vi "RxTx.vi"(0 "State-machine Local Variables":T1={"Message"="", "Homed?"=FALSE, "NextState"=enum."Timeout", "G.Load"=0.0, "G.Position"=0.0, "Load#"=0, "[G.Loads]"=[], "[TotalLoads]"=[], "[Errors]"=[], "ZeroWait"=0, "Results"=[], "DwellWait"=FALSE, "Test Result"=FALSE, "[CondyleLoads]"=[], "[Max]"=[], "[Min]"=[], "Valid String?"=FALSE, "ScanTime"=timestamp(0 s since 1904-01-01), "ScannedString"="", "LabelDevID"=0, "MfgDate"=timestamp(0 s since 1904-01-01), "[EEPROM Cmds]"=[], "[CalData]"=[], "[A/Ds]"=[], "[A/Dmax]"=[], "[A/Dmin]"=[], "BattMax"=0.0, "BattMin"=0.0, "DwellTime"=2000, "PendingDeviceType"="", "Zero G.load"=0.0, "GAINC Value"="", "Programming Step"=enum."Load EEPROM", "Front Panel Program?"=FALSE, "Final Program?"=FALSE, "PCB Score"=100, "AssyScore"=100, "Pass/Fail #"="", "Result String"="", "Programming Mode"=enum."Initial Program", "Angle Test Step"=enum."Initialize", "Accel Values"=[], "Shutdown Counter"=0, "V1"=0, "V2"=0, "V3"=0, "V4"=0, "EEPROM Data"=[], "Counter"=0, "Page#"=0, "Timer"=timestamp(0 s since 1904-01-01), "Use Mark10?"=FALSE, "Eng-Result#"=0, "DUT Serial #"=0, "Scroll Message?"=FALSE, "Clear Message"=FALSE, "Batt Test Step "=enum."Initialize", "RXTX Window Found?"=FALSE, "Shutdown First Call?"=FALSE, "A2 Delay (msec)"=500, "Support Script"={"Script #"="", "Script Revision"="", "[OEMs]"=[], "[[DeviceTypes]]"=[], "[[DeviceTypesVals]]"=[], "[[List of Errors]]"=[], "Default GAINC"="", "[[ASICtrims]]"=[], "ID For Echo"="", "Condyle A CalFactor"=100, "Condyle B CalFactor"=100, "[OEMs Prefix]"=[], "Packet ID 18"="", "[[Force Table Load Test]]"=[], "[[Force Table AccurTest]]"=[]}, "Serial Table"={"Serial File Path"=path "", "[[Serial Lookup Table]]"=[], "Serial Device Info"=[], "Valid Serial?"=FALSE}, "Target Information"={"Target Brand"="", "Target DeviceType"="", "Target Serial#"=100, "Target Lot#"=0, "Target DevID"=0, "Target Channel"=5}, "Operator"="", "COM Port"="", "Config Path"=path "", "Tx Array"=[], "DUT Parameters"={"Channel"=0, "DeviceID"=0, "Script Rev"=0, "Month"=0, "Day"=0, "Year"=0, "Lot#"=0, "V1"=0, "V2"=0, "V3"=0, "V4"=0, "MFG"=0, "Cal FactorA 10"=0, "Cal FactorB 10  "=0, "Cal FactorA 16"=0, "Cal FactorB 16"=0, "ASICtrim"=[], "TmpChan"=0, "GAINC"="", "Brand"="", "Device"="", "Serial #"=0, "Batt310"=0, "Batt 280"=0}, "FTS Main?"=FALSE, "Loading"={"[Forces]"=[], "[Dwell]"=[], "Loading Step"=enum."Initialize Test"}, "Software Version"="", "Correction Factor"="", "Second Load Test"=FALSE, "Acc Loads"=[], "Mark10 Config"={"H2S%"=[80.0, 85.0, 90.0, 95.0, 100.0], "H2S Speed"=[12.0, 8.0, 6.0, 4.0, 2.0], "H to S"=2.0, "Home Speed"=1.0, "LoadWin"=0.0, "Load Speed"=0.0, "PID"={"Kp"=0.04, "Kd"=0.005001, "Ki"=2.9999999999999923e-05}}, "Channels"={"Transceiver Ch"=5, "Operating Ch"=5, "Start Ch"=0}, "Channel EEPROM"=[], "Load Notes"=[], "Engr Log?"=FALSE, "Time"=[], "Program Retry"=FALSE, "Operator Channel"="", "Target Channel "="", "New Data Program"=FALSE, "NFHU Pass?"=FALSE, "Cycle Number"=0, "Cal Cycle#"=0, "[Avg G.Loads] "=[], "[Avg A/Ds] "=[], "Cal Retry?"=FALSE, "[Total A/Ds]  "=[], "Cycle Num LA"=0, "LA Cycle# "=0, "Shim Num"=0, "Shim#  "=0, "Angle Test?"=FALSE} {"Mark10 Config"."PID"."Ki" min=0.0 max=200.0 format="%.6f"; "Mark10 Config"."PID"."Kd" min=0.0 max=200.0 format="%.6f"; "Mark10 Config"."PID"."Kp" min=0.0 max=200.0 format="%.6f"; "DUT Parameters"."ASICtrim" format="%02x"}, 2 "[TxData]":u8[](array[numeric]), 5 "error in (no error)":errorcluster, 9 "Action":T15) -> (8 "NoData?":bool, 10 "Blank?":bool, 11 "return type":i32, 14 "[Raw RxData]":u8[](array[numeric]), 15 "Alive?":bool, 16 "Stop?":bool, 17 "NewData?":bool, 18 "DUT Serial Number":u32, 19 "error out":errorcluster)   [LabVIEW 2015]
uses:
  XceiverStates.ctl
  Controls/LocalVars.ctl
  Controls/Gen2 FT states.ctl
  Controls/Iniial Device Programming.ctl
  SubVI/ProgramStageControl.ctl
  Controls/Batt Cap Steps.ctl
  Controls/Support Script.ctl
  Controls/Serial Table.ctl
  Controls/Device Information.ctl
  Controls/InfoPacket.ctl
  Controls/Loading.ctl
  Controls/Load Step.ctl
  Controls/Mark10 Config.ctl
  Controls/PID parameters.ctl
  Controls/Channels.ctl
  Controls/Gen2 FT Globals.vi
  data/SiUSBXp.dll
panel:
  out "Handle":u32
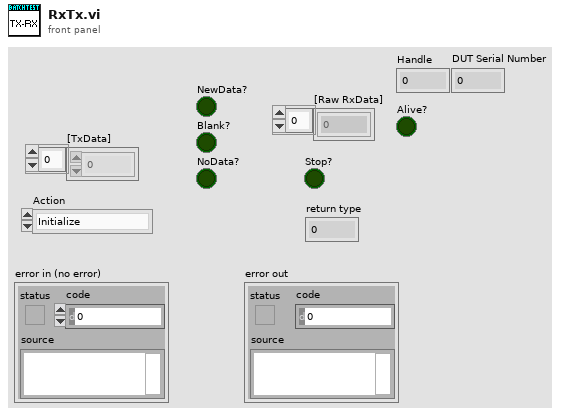
[diagram p1: front panel]
types:
  T1 = typedef "LocalVars.ctl" = cluster{"Message":string, "Homed?":bool, "NextState":T2, "G.Load":dbl, "G.Position":dbl, "Load#":i32, "[G.Loads]":dbl[], "[TotalLoads]":dbl[], "[Errors]":dbl[][], "ZeroWait":u32, "Results":dbl[], "DwellWait":bool, "Test Result":bool, "[CondyleLoads]":dbl[][], "[Max]":dbl[], "[Min]":dbl[], "Valid String?":bool, "ScanTime":timestamp, "ScannedString":string, "LabelDevID":u32, "MfgDate":timestamp, "[EEPROM Cmds]":u8[][], "[CalData]":u8[][], "[A/Ds]":dbl[][], "[A/Dmax]":dbl[], "[A/Dmin]":dbl[], "BattMax":dbl, "BattMin":dbl, "DwellTime":i32, "PendingDeviceType":string, "Zero G.load":dbl, "GAINC Value":string, "Programming Step":T3, "Front Panel Program?":bool, "Final Program?":bool, "PCB Score":i32, "AssyScore":i32, "Pass/Fail #":string, "Result String":string, "Programming Mode":T4, "Angle Test Step":enum16{"Initialize", "Get X", "Get Y", "Get Z", "Next Test"}, "Accel Values":dbl[][], "Shutdown Counter":u32, "V1":i32, "V2":i32, "V3":i32, "V4":i32, "EEPROM Data":i32[][], "Counter":i32, "Page#":i32, "Timer":timestamp, "Use Mark10?":bool, "Eng-Result#":u32, "DUT Serial #":i32, "Scroll Message?":bool, "Clear Message":bool, "Batt Test Step ":T5, "RXTX Window Found?":bool, "Shutdown First Call?":bool, "A2 Delay (msec)":i16, "Support Script":T6, "Serial Table":T7, "Target Information":T8, "Operator":string, "COM Port":string, "Config Path":path, "Tx Array":u8[], "DUT Parameters":T9, "FTS Main?":bool, "Loading":T10, "Software Version":string, "Correction Factor":string, "Second Load Test":bool, "Acc Loads":dbl[][], "Mark10 Config":T12, "Channels":T14, "Channel EEPROM":i32[][], "Load Notes":string[], "Engr Log?":bool, "Time":timestamp[], "Program Retry":bool, "Operator Channel":string, "Target Channel ":string, "New Data Program":bool, "NFHU Pass?":bool, "Cycle Number":i32, "Cal Cycle#":i32, "[Avg G.Loads] ":dbl[], "[Avg A/Ds] ":dbl[][], "Cal Retry?":bool, "[Total A/Ds]  ":dbl[][], "Cycle Num LA":i32, "LA Cycle# ":i32, "Shim Num":i32, "Shim#  ":i32, "Angle Test?":bool}
  T2 = typedef "Gen2 FT states.ctl" = enum16{"---------SETUP-------", "Initialization", "Read Support Data", "Initialize Mark-10", "Initialize Transceiver", "------UTILITIES------", "Change DUT Channel", "Find RxTx Window", "Reset Device", "Scan Channels", "Read Serial Lookup", "Shutdown Device", "ESTOP", "--------USER---------", "Timeout", "-----PROGRAM-----", "Program Device", "------MARK10--------", "Go Home", "MoveUp", "MoveDown", "Goto Load", "Goto Position", "Stop Motor", "---------TESTS--------", "Start Test", "Angle Test", "Load Test", "Load Accuracy Test", "Battery Test", "------RESULTS-------", "End Test", "Display Result", "--------EXIT--------", "Exit"}
  T3 = typedef "Iniial Device Programming.ctl" = enum16{"Load EEPROM", "Send First A1", "Send EEPROM", "Send A1", "Check EEPROM Echo", "Verify transmission", "Programming Successful", "Programming Failed"}
  T4 = typedef "ProgramStageControl.ctl" = enum16{"Initial Program", "GainC", "Scales"}
  T5 = typedef "Batt Cap Steps.ctl" = enum16{"Initialize", "Collect 2.8 Volts", "Collect 3.1 Volts", "Check Results"}
  T6 = typedef "Support Script.ctl" = cluster{"Script #":string, "Script Revision":string, "[OEMs]":string[], "[[DeviceTypes]]":string[][], "[[DeviceTypesVals]]":u16[][], "[[List of Errors]]":string[][], "Default GAINC":string, "[[ASICtrims]]":u8[][], "ID For Echo":string, "Condyle A CalFactor":i32, "Condyle B CalFactor":i32, "[OEMs Prefix]":string[], "Packet ID 18":string, "[[Force Table Load Test]]":dbl[][], "[[Force Table AccurTest]]":dbl[][]}
  T7 = typedef "Serial Table.ctl" = cluster{"Serial File Path":path, "[[Serial Lookup Table]]":string[][], "Serial Device Info":string[], "Valid Serial?":bool}
  T8 = typedef "Device Information.ctl" = cluster{"Target Brand":string, "Target DeviceType":string, "Target Serial#":i32, "Target Lot#":u32, "Target DevID":u32, "Target Channel":u8}
  T9 = typedef "InfoPacket.ctl" = cluster{"Channel":u8, "DeviceID":u32, "Script Rev":u8, "Month":u8, "Day":u8, "Year":u8, "Lot#":u32, "V1":u16, "V2":u16, "V3":u16, "V4":u16, "MFG":u8, "Cal FactorA 10":u8, "Cal FactorB 10  ":u8, "Cal FactorA 16":u8, "Cal FactorB 16":u8, "ASICtrim":u8[], "TmpChan":u8, "GAINC":string, "Brand":string, "Device":string, "Serial #":u64, "Batt310":u16, "Batt 280":u16}
  T10 = typedef "Loading.ctl" = cluster{"[Forces]":dbl[], "[Dwell]":dbl[], "Loading Step":T11}
  T11 = typedef "Load Step.ctl" = enum16{"Initialize Test", "Go Home", "Detect Dev Surface", "Wait to zero Device", "Zero Device", "Do Test", "Test Result"}
  T12 = typedef "Mark10 Config.ctl" = cluster{"H2S%":dbl[], "H2S Speed":dbl[], "H to S":dbl, "Home Speed":dbl, "LoadWin":dbl, "Load Speed":dbl, "PID":T13}
  T13 = typedef "PID parameters.ctl" = cluster{"Kp":dbl, "Kd":dbl, "Ki":dbl}
  T14 = typedef "Channels.ctl" = cluster{"Transceiver Ch":u8, "Operating Ch":u8, "Start Ch":u8}
  T15 = typedef "XceiverStates.ctl" = enum16{"Initialize", "Rx", "Tx", "Raw Mode", "Clear Buffer", "ClearEcho", "Read Buffer", "Close"}
  T16 = cluster{"Handle":u32, "TempRxData":u8[], "OffTimer":u32, "Echo?":bool, "NoData?":bool, "Alive?":bool, "Counter":u32}
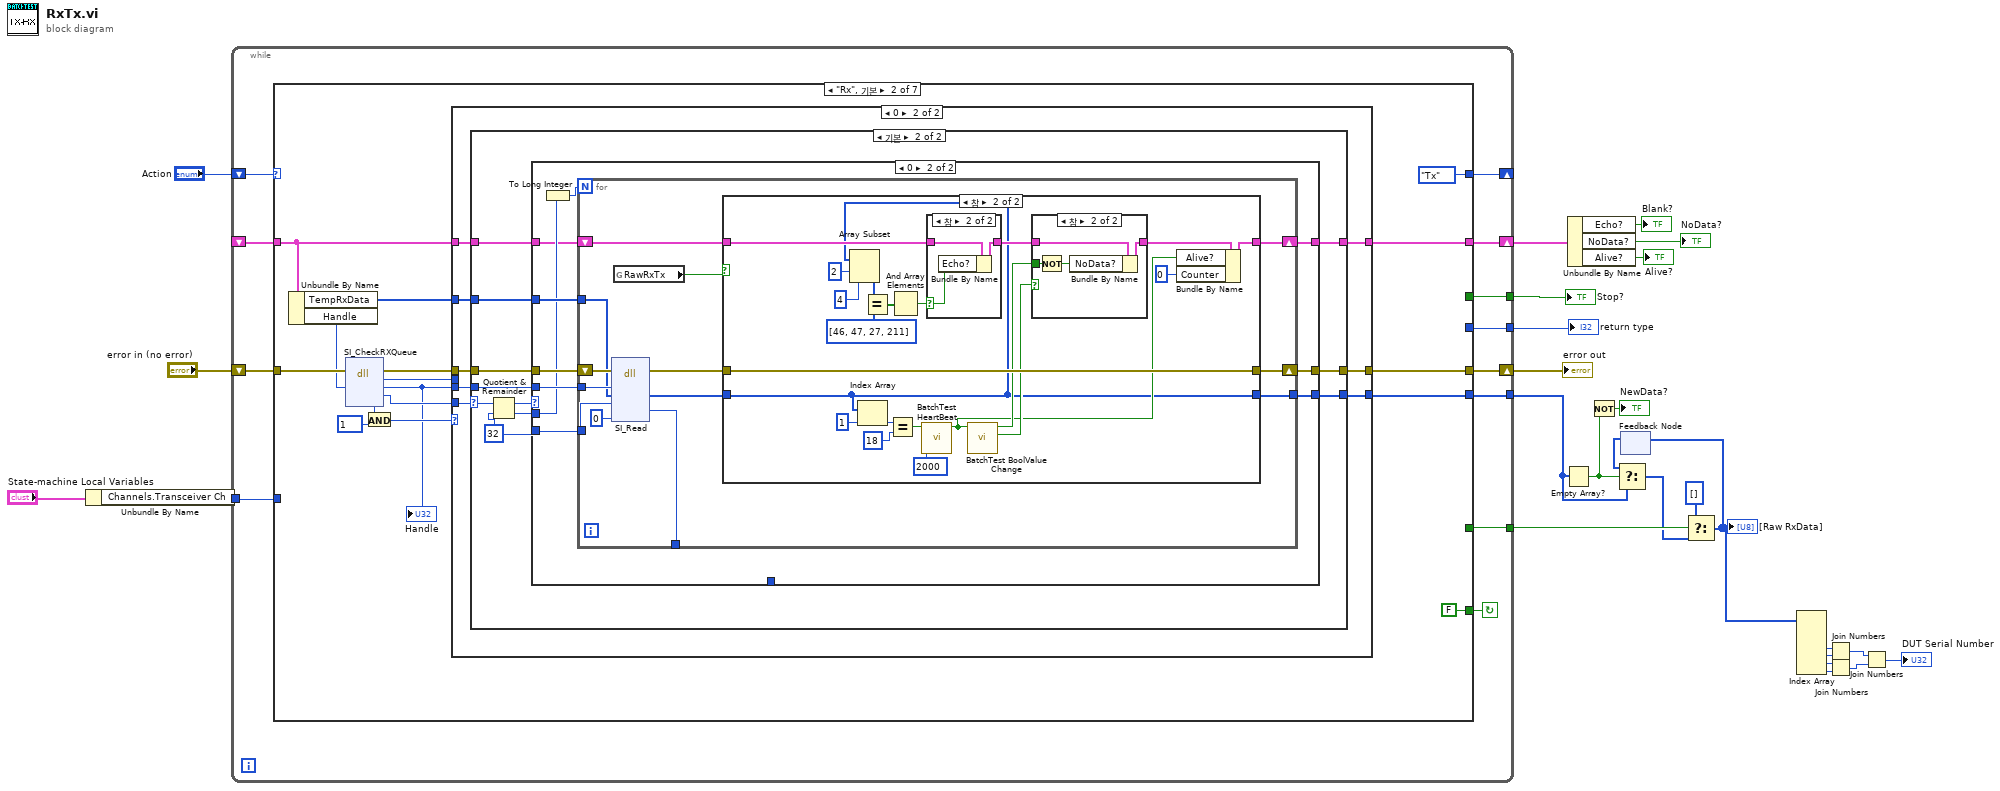
[diagram p0: block diagram]
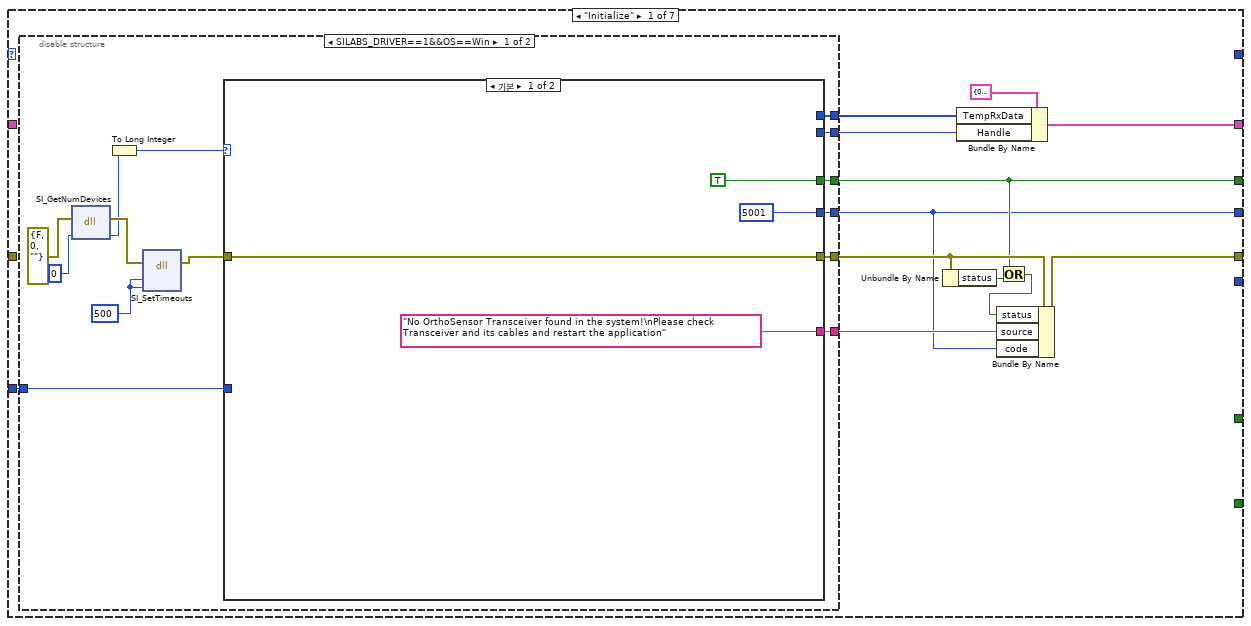
[diagram p2: hidden frame]
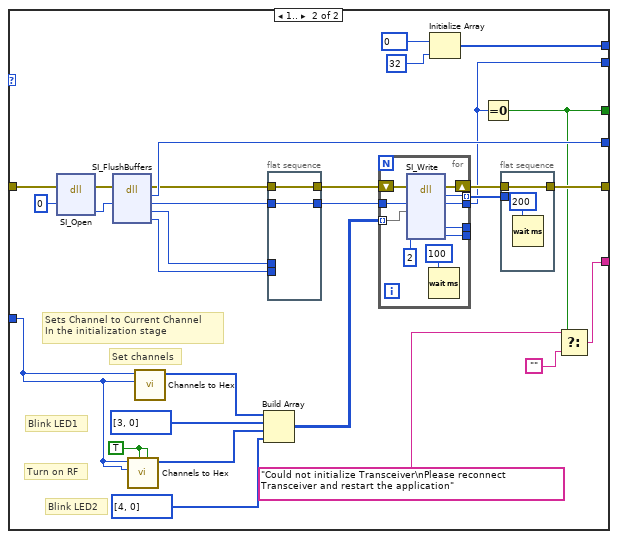
[diagram p3: hidden frame]
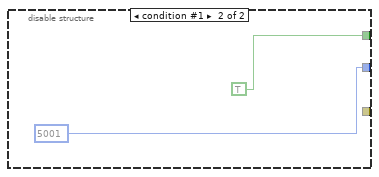
[diagram p4: hidden frame]
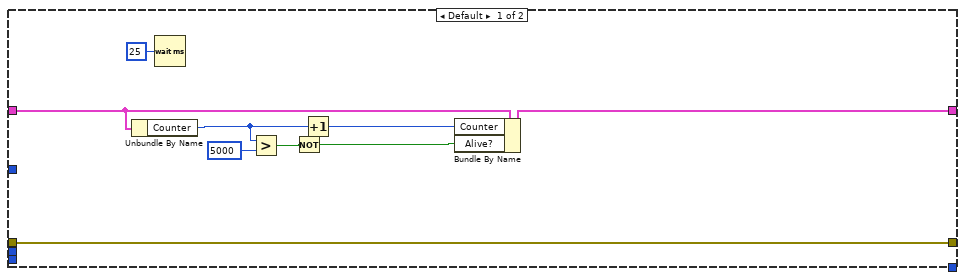
[diagram p5: hidden frame]
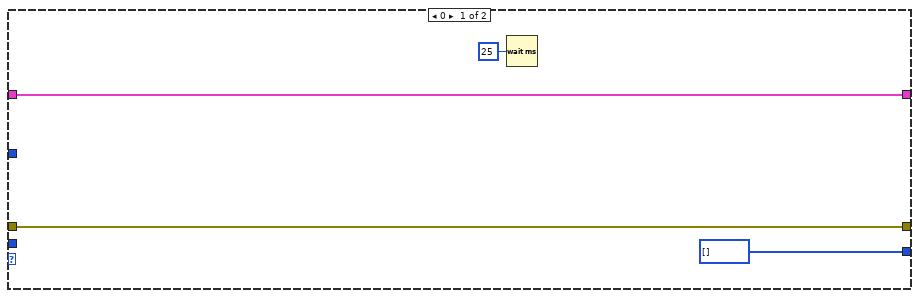
[diagram p6: hidden frame]
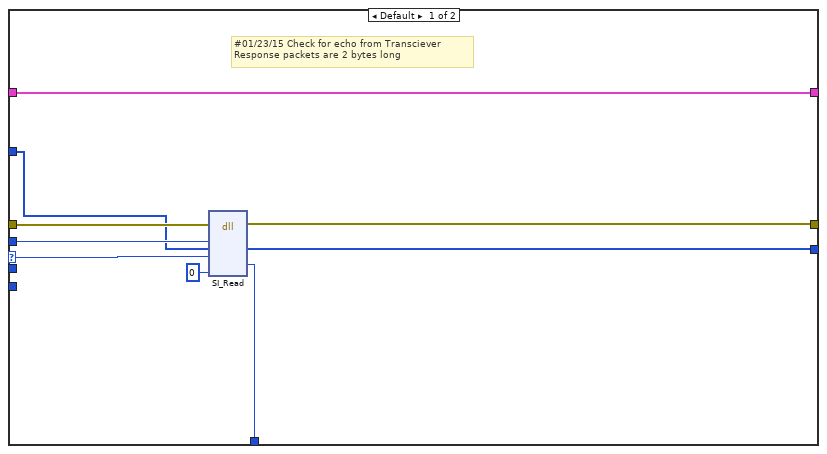
[diagram p7: hidden frame]
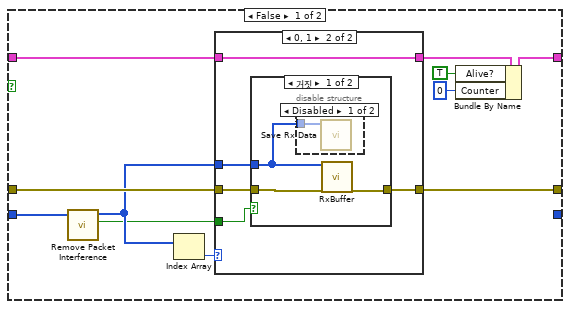
[diagram p8: hidden frame]
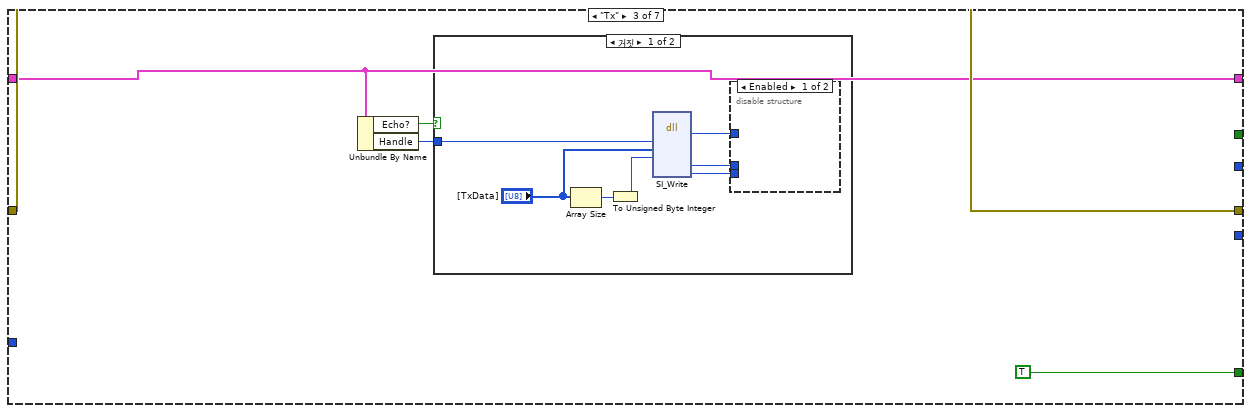
[diagram p14: hidden frame]
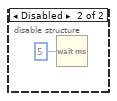
[diagram p15: hidden frame]
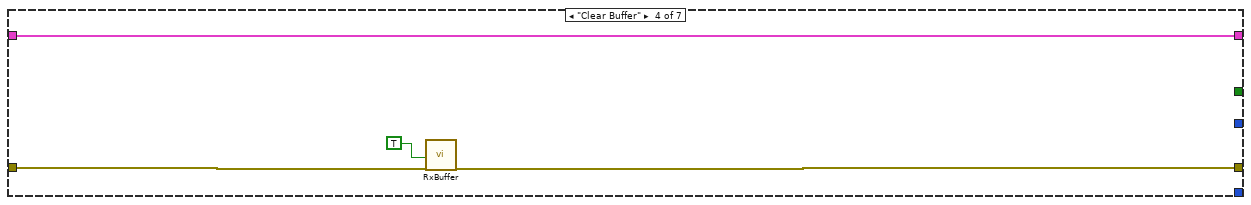
[diagram p17: hidden frame]
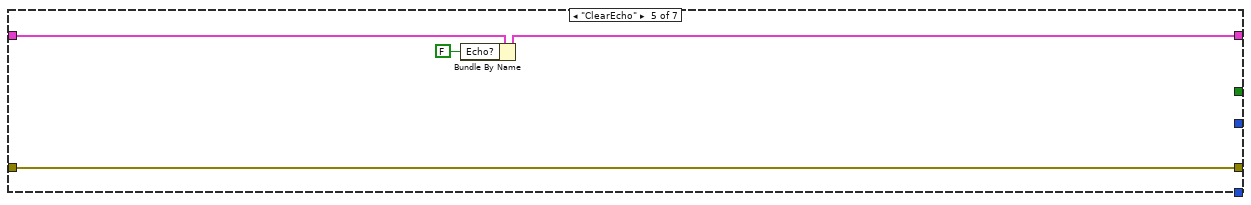
[diagram p18: hidden frame]
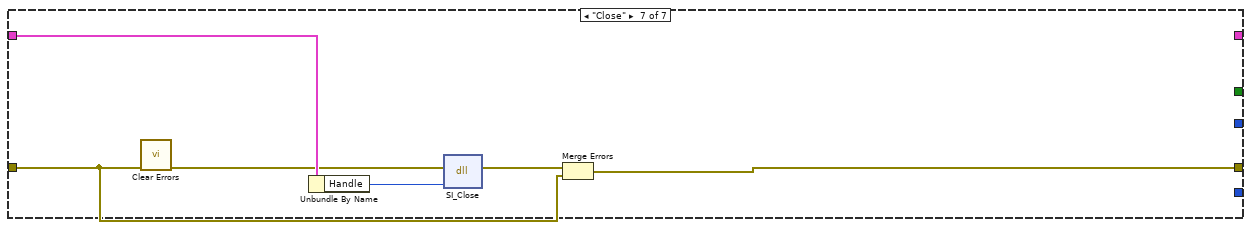
[diagram p20: hidden frame]
diagram:
  n1 = Unbundle By Name("State-machine Local Variables") -> ("Channels.Transceiver Ch"=w9:u8)
  n2 = while {
    shift-right: [w38] -> w14
    shift-left: _ -> [w37]
    shift-right: [w35] -> w26
    shift-left: "error in (no error)" -> [w36]
    tunnel: [w34] -> w23
    tunnel: [w32] -> w22
    shift-right: [w30] -> _
    shift-left: "Action" -> [w33]
    tunnel: [w29] -> w19
    tunnel: [w28] -> w17
    tunnel: w9 -> [w27]
    stop <- w31 continue-if-true
    n3 = case shown="\"Rx\", 기본" w33 {
      tunnel: [w49 w117 w250 w263 w265 w269 _] -> w38
      tunnel: w37 -> [_ w118 w250 w263 w267 w269 w274]
      tunnel: w36 -> [_ w128 w251 w262 w266 w268 w270]
      tunnel: [w45 w129 w251 w261 w266 w268 w271] -> w35
      tunnel: [w40 _ _ _ _ _ _] -> w34
      tunnel: [w42 _ _ _ _ _ _] -> w32
      tunnel: [_ FALSE ("Shutdown?") _ _ _ _ _] -> w31
      tunnel: [_ XceiverStates."Tx" ("Action") _ _ _ _ _] -> w30
      tunnel: [_ w115 _ _ _ _ _] -> w29
      tunnel: [_ _ TRUE _ _ _ _] -> w28
      tunnel: w27 -> [w39 _ _ _ _ _ _]
      frame "Initialize" {
        n4 = disable-structure shown="SILABS_DRIVER==1&&OS==Win" {
          disable-tunnel: [w58 _] -> w48
          disable-tunnel: [w57 _] -> w47
          disable-tunnel: [w55 _] -> w46
          disable-tunnel: [w54 TRUE] -> w42
          disable-tunnel: [w53 _] -> w41
          disable-tunnel: [w52 5001 ("return type")] -> w40
          disable-tunnel: w39 -> [w51 _]
          frame condition #0 (active) {
            w60 = u32 500 ("WriteTimeout")
            n5 = dll-call lib="D:/KSY_Work/LabVIEW/GEN3 FTS Software(FTS Test)/Orthosensor FTS/data/SiUSBXp.dll" fn="SI_GetNumDevices"(error in=errorcluster {"status"=FALSE, "code"=0, "source"=""} ("error in (no error)"), "NumDevices"=u32 0) -> (error out=w62:errorcluster, "NumDevices"=w59:u32)  [unwired: 3 in, 1 out]
            n6 = To Long Integer(number=w59) -> (32bit integer=w56:i32)
            n7 = dll-call lib="D:/KSY_Work/LabVIEW/GEN3 FTS Software(FTS Test)/Orthosensor FTS/data/SiUSBXp.dll" fn="SI_SetTimeouts"(error in=w62, "ReadTimeout"=w60, "WriteTimeout"=w60) -> (error out=w63:errorcluster)  [unwired: 5 in, 1 out]
            n8 = case shown="기본" w56 {
              tunnel: w63 -> [w68 w97]
              tunnel: [w68 w89] -> w55
              tunnel: [_ w76] -> w58
              tunnel: [5001 ("return type") w85] -> w52
              tunnel: [_ w78] -> w57
              tunnel: [TRUE w74] -> w54
              tunnel: ["No OrthoSensor Transceiver found in the system!\nPlease check Transceiver and its cables and restart the application" w75] -> w53
              tunnel: w51 -> [_ w69]
              frame Default {
              }
              frame 1.. {
                w88 = TRUE ("RF Chip0 Enable")
                # "Sets Channel to Current Channel\nIn the initialization stage"
                # "Blink LED2"
                # "Turn on RF"
                # "Blink LED1"
                # "Set channels"
                n9 = dll-call lib="D:/KSY_Work/LabVIEW/GEN3 FTS Software(FTS Test)/Orthosensor FTS/data/SiUSBXp.dll" fn="SI_Open"(error in=w97, "DeviceNum"=u32 0) -> (error out=w83:errorcluster, "Handle"=w84:u32)  [unwired: 5 in, 1 out]
                n10 = dll-call lib="D:/KSY_Work/LabVIEW/GEN3 FTS Software(FTS Test)/Orthosensor FTS/data/SiUSBXp.dll" fn="SI_FlushBuffers"(error in=w83, "Handle"=w84) -> (error out=w71:errorcluster, "return type"=w85:i32, "Handle"=w70:u32, "NumBytesInQueue"=w82:u32, "QueueStatus"=w81:u32)  [unwired: 4 in, 1 out]
                n11 = call "Channels to Hex.vi"("RF Chip1 Enable"=w88, "RF Chip0 Enable"=w88, "RF Chip0 Channel"=w69, "RF Chip1 Channel"=w69) -> ("Command"=w91:u8[])  [unwired: 7 in]
                n12 = call "Channels to Hex.vi"("RF Chip0 Channel"=w69, "RF Chip1 Channel"=w69) -> ("Command"=w94:u8[])  [unwired: 9 in]
                n13 = Build Array(w94, u8[] [3, 0], w91, u8[] [4, 0]) -> (w93:u8[][])
                n14 = flat-sequence {
                  tunnel: w71 -> [w111]
                  tunnel: [w111] -> w95
                  tunnel: w70 -> [w110]
                  tunnel: [w110] -> w96
                  tunnel: w82 -> [_]
                  tunnel: w81 -> [_]
                  frame #0 {
                  }
                }
                n15 = for {
                  tunnel: w96 -> [w107]
                  shift-right: [w108] -> w87
                  shift-left: w95 -> [w109]
                  tunnel: [w105] -> _
                  tunnel: [w104] -> _
                  tunnel: [w103] -> w76
                  tunnel: [w102] -> w86 mode=indexing
                  tunnel: w93 -> [w101] mode=indexing
                  n16 = dll-call lib="D:/KSY_Work/LabVIEW/GEN3 FTS Software(FTS Test)/Orthosensor FTS/data/SiUSBXp.dll" fn="SI_Write"(error in=w109, "Handle"=w107, "Buffer"=w101, "NumBytesToWrite"=u8 2) -> (error out=w108:errorcluster, "return type"=w102:u8, "Handle"=w103:u32, "NumBytesWritten"=w105:u8, "o"=w104:u32)  [unwired: 6 in, 1 out]
                  n17 = Wait (ms)(milliseconds to wait=u32 100) -> ()  [unwired: 1 out]
                }
                n18 = Initialize Array(u8 0, 32 ("dimension size")) -> (w78:u8[])
                n19 = Equal To 0?(x=w76) -> (x = 0?=w74:bool)
                n20 = flat-sequence {
                  tunnel: w87 -> [w99]
                  tunnel: [w99] -> w89
                  tunnel: w86 -> [_]
                  frame #0 {
                    n21 = Wait (ms)(milliseconds to wait=u32 200) -> ()  [unwired: 1 out]
                  }
                }
                n22 = Select(t="Could not initialize Transceiver\nPlease reconnect Transceiver and restart the application", s=w74, f="") -> (s? t:f=w75:string)
              }
            }
          }
          frame condition #1 {
          }
        }
        n23 = Unbundle By Name(w46) -> ("status"=w43:bool)
        n24 = Bundle By Name(cluster=T16 {"Handle"=0, "TempRxData"=[], "OffTimer"=0, "Echo?"=FALSE, "NoData?"=FALSE, "Alive?"=FALSE, "Counter"=0}, "TempRxData"=w47, "Handle"=w48) -> (w49:T16)
        n25 = Or(x=w42, y=w43) -> (x .or. y?=w44:bool)
        n26 = Bundle By Name(cluster=w46, "status"=w44, "source"=w41, "code"=w40) -> (w45:errorcluster)
      }
      frame "Rx", Default {
        n27 = Unbundle By Name(w118) -> ("TempRxData"=w126:u8[], "Handle"=w127:u32)
        n28 = dll-call lib="D:/KSY_Work/LabVIEW/GEN3 FTS Software(FTS Test)/Orthosensor FTS/data/SiUSBXp.dll" fn="SI_CheckRXQueue"(error in=w128, "Handle"=w127) -> (error out=w120:errorcluster, "return type"=w119:i32, "Handle"=w121:u32, "NumBytesInQueue"=w122:u32, "QueueStatus"=w125:u32)  [unwired: 4 in, 1 out]
        "Handle" <- w121
        n29 = And(x=w125, y=u32 1) -> (x .and. y?=w123:u32)
        n30 = case shown="0" w123 {
          tunnel: w122 -> [_ w146]
          tunnel: w121 -> [_ w145]
          tunnel: w120 -> [w138 w144]
          tunnel: [w138 w143] -> w129
          tunnel: w119 -> [_ _]
          tunnel: w126 -> [_ w142]
          tunnel: w118 -> [w136 w141]
          tunnel: [w135 w140] -> w117
          tunnel: [_ w139] -> w115
          frame Default {
            n31 = Unbundle By Name(w136) -> ("Counter"=w133:u32)
            n32 = Wait (ms)(milliseconds to wait=u32 25) -> ()  [unwired: 1 out]
            n33 = Greater?(x=w133, y=u32 5000) -> (0:w131:bool)
            n34 = Not(x=w131) -> (.not. x?=w130:bool)
            n35 = Increment(x=w133) -> (x+1=w134:u32)
            n36 = Bundle By Name(cluster=w136, "Counter"=w134, "Alive?"=w130) -> (w135:T16)
          }
          frame 0 {
            n37 = case shown="기본" w146 {
              selector: w146 -> [_ w158]
              tunnel: w145 -> [_ w161]
              tunnel: w144 -> [w150 w160]
              tunnel: [w150 w159] -> w143
              tunnel: w142 -> [_ w157]
              tunnel: w141 -> [w148 w153]
              tunnel: [w148 w152] -> w140
              tunnel: [u8[] [] ("Buffer") w151] -> w139
              frame 0 {
                n38 = Wait (ms)(milliseconds to wait=u32 25) -> ()  [unwired: 1 out]
              }
              frame Default {
                w155 = u32 32 ("y")
                n39 = Quotient & Remainder(x=w158, y=w155) -> (x-y*floor(x/y)=w156:u32, floor(x/y)=w154:u32)
                n40 = case shown="0" w156 {
                  selector: w156 -> [w168 _]
                  tunnel: w161 -> [w169 w180]
                  tunnel: w160 -> [w170 w179]
                  tunnel: [w162 w178] -> w159
                  tunnel: [w164 _] -> _
                  tunnel: w157 -> [w166 w177]
                  tunnel: w155 -> [_ w176]
                  tunnel: w154 -> [_ w175]
                  tunnel: w153 -> [w167 w173]
                  tunnel: [w167 w172] -> w152
                  tunnel: [w163 w171] -> w151
                  frame Default {
                    # "#01/23/15 Check for echo from Transciever\nResponse packets are 2 bytes long"
                    n41 = dll-call lib="D:/KSY_Work/LabVIEW/GEN3 FTS Software(FTS Test)/Orthosensor FTS/data/SiUSBXp.dll" fn="SI_Read"(error in=w170, "Handle"=w169, "Buffer"=w166, "NumBytesToRead"=w168, "o"=u32 0) -> (error out=w162:errorcluster, "Buffer"=w163:u8[], "NumBytesReturned"=w164:u32)  [unwired: 7 in, 1 out]
                  }
                  frame 0 {
                    n42 = To Long Integer(number=w175) -> (32bit integer=w174:i32)
                    n43 = for {
                      N: w174 -> [_]
                      tunnel: w180 -> [w193]
                      tunnel: w177 -> [w190]
                      tunnel: w176 -> [w189]
                      shift-right: [w187] -> w178
                      shift-left: w179 -> [w192]
                      tunnel: [w186] -> _
                      shift-right: [w184] -> w172
                      shift-left: w173 -> [w185]
                      tunnel: [w183] -> w171
                      n44 = dll-call lib="D:/KSY_Work/LabVIEW/GEN3 FTS Software(FTS Test)/Orthosensor FTS/data/SiUSBXp.dll" fn="SI_Read"(error in=w192, "Handle"=w193, "Buffer"=w190, "NumBytesToRead"=w189, "o"=u32 0) -> (error out=w188:errorcluster, "Buffer"=w181:u8[], "NumBytesReturned"=w186:u32)  [unwired: 7 in, 1 out]
                      n45 = global read "Gen2 FT Globals.vi" "RawRxTx"() -> (w182:bool)
                      n46 = case shown="참" w182 {
                        tunnel: w181 -> [w196 w217]
                        tunnel: w188 -> [w203 w236]
                        tunnel: [w202 w236] -> w187
                        tunnel: w185 -> [w201 w237]
                        tunnel: [w199 w220] -> w184
                        tunnel: [_ w217] -> w183
                        frame False {
                          n47 = call "Remove Packet Interference.vi"("Buffer in"=w196) -> ("Filtered?"=w194:bool, "Buffer out"=w195:u8[])  [unwired: 9 in]
                          n48 = Index Array(array=w195) -> (element=w204:u8)  [unwired: 1 in]
                          n49 = case shown="0, 1" w204 {
                            tunnel: w195 -> [_ w209]
                            tunnel: w203 -> [w205 w211]
                            tunnel: [w205 w208] -> w202
                            tunnel: w201 -> [w206 w210]
                            tunnel: [w206 w210] -> w200
                            tunnel: w194 -> [_ w207]
                            frame Default {
                            }
                            frame 0, 1 {
                              n50 = case shown="거짓" w207 {
                                tunnel: w211 -> [w214 w216]
                                tunnel: w209 -> [w213 _]
                                tunnel: [w212 w216] -> w208
                                frame False {
                                n51 = disable-structure shown="Disabled" {
                                disable-tunnel: w213 -> [w215 _]
                                frame Disabled {
                                n52 = call "Save Rx Data.vi"("Buffer in"=w215) -> ()  [unwired: 11 in]
                                }
                                frame Enabled {
                                }
                                }
                                n53 = call "RxBuffer.vi"("RxData"=w213, "error in (no error)"=w214) -> ("error out"=w212:errorcluster)  [unwired: 6 in, 11 out]
                                }
                                frame True {
                                # "Filter Out\nCross talk"
                                }
                              }
                            }
                          }
                          n54 = Bundle By Name(cluster=w200, "Alive?"=TRUE, "Counter"=u32 0) -> (w199:T16)
                        }
                        frame True {
                          n55 = Array Subset(array=w217, index=2, length=4) -> (w232:u8[])
                          n56 = Index Array(array=w217, index=1) -> (element=w227:u8)
                          n57 = Equal?(x=w232, y=u8[] [46, 47, 27, 211] ("RawTx")) -> (x = y?=w233:bool[])
                          n58 = Equal?(x=w227, y=u8 18) -> (x = y?=w225:bool)
                          n59 = And Array Elements(Boolean array=w233) -> (logical AND=w230:bool)
                          n60 = call "BatchTest HeartBeat.vi"("MaxTime"=u32 2000, "Value In"=w225) -> ("Alive?"=w219:bool)  [unwired: 8 in, 1 out]
                          n61 = case shown="참" w230 {
                            selector: w230 -> [_ w244]
                            tunnel: w237 -> [w243 w246]
                            tunnel: [w243 w245] -> w228
                            frame False {
                            }
                            frame True {
                              n62 = Bundle By Name(cluster=w246, "Echo?"=w244) -> (w245:T16)
                            }
                          }
                          n63 = call "BatchTest BoolValue Change.vi"("Value In"=w219) -> ("Value Changed?"=w223:bool, "Value Out"=w222:bool)  [unwired: 7 in, 2 out]
                          n64 = case shown="참" w223 {
                            tunnel: w228 -> [w238 w242]
                            tunnel: [w238 w241] -> w221
                            tunnel: w222 -> [_ w240]
                            frame False {
                            }
                            frame True {
                              n65 = Not(x=w240) -> (.not. x?=w239:bool)
                              n66 = Bundle By Name(cluster=w242, "NoData?"=w239) -> (w241:T16)
                            }
                          }
                          n67 = Bundle By Name(cluster=w221, "Alive?"=w219, "Counter"=u32 0) -> (w220:T16)
                        }
                      }
                    }
                  }
                }
              }
            }
          }
        }
      }
      frame "Tx" {
        n68 = Unbundle By Name(w250) -> ("Echo?"=w247:bool, "Handle"=w248:u32)
        n69 = case shown="거짓" w247 {
          tunnel: w248 -> [w258 _]
          frame False {
            n70 = Array Size(array="[TxData]") -> (size(s)=w257:i32)
            n71 = To Unsigned Byte Integer(number=w257) -> (unsigned 8bit integer=w256:u8)
            n72 = dll-call lib="D:/KSY_Work/LabVIEW/GEN3 FTS Software(FTS Test)/Orthosensor FTS/data/SiUSBXp.dll" fn="SI_Write"("Handle"=w258, "Buffer"="[TxData]", "NumBytesToWrite"=w256) -> ("return type"=w254:u8, "NumBytesWritten"=w253:u8, "o"=w252:u32)  [unwired: 8 in, 2 out]
            n73 = disable-structure shown="Enabled" {
              disable-tunnel: w254 -> [_ _]
              disable-tunnel: w253 -> [_ _]
              disable-tunnel: w252 -> [_ _]
              frame Enabled {
              }
              frame Disabled {
                n74 = Wait (ms)(milliseconds to wait=u32 5) -> ()  [unwired: 1 out]
              }
            }
          }
          frame True {
          }
        }
      }
      frame "Clear Buffer" {
        n75 = call "RxBuffer.vi"("Clear?"=TRUE, "error in (no error)"=w262) -> ("error out"=w261:errorcluster)  [unwired: 6 in, 11 out]
      }
      frame "ClearEcho" {
        n76 = Bundle By Name(cluster=w267, "Echo?"=FALSE ("Blank?")) -> (w265:T16)
      }
      frame "Read Buffer" {
      }
      frame "Close" {
        n77 = call <vilib>:"Clear Errors.vi"("error in (no error)"=w270) -> ("error out"=w273:errorcluster)  [unwired: 5 in, 1 out]
        n78 = Unbundle By Name(w274) -> ("Handle"=w272:u32)
        n79 = dll-call lib="D:/KSY_Work/LabVIEW/GEN3 FTS Software(FTS Test)/Orthosensor FTS/data/SiUSBXp.dll" fn="SI_Close"(error in=w273, "Handle"=w272) -> (error out=w275:errorcluster)  [unwired: 4 in, 1 out]
        n80 = Merge Errors(w275, w270) -> (w271:errorcluster)
      }
    }
  }
  "error out" <- w26
  "return type" <- w23
  "Stop?" <- w22
  n81 = Empty Array?(array=w19) -> (empty?=w21:bool)
  n82 = Unbundle By Name(w14) -> ("Echo?"=→"Blank?":bool, "NoData?"=→"NoData?":bool, "Alive?"=→"Alive?":bool)
  n83 = Not(x=w21) -> (.not. x?=→"NewData?":bool)
  n84 = feedback #1() -> (w20:u8[])  [unwired: 1 in]
  n85 = Select(t=w20, s=w21, f=w19) -> (s? t:f=w15:u8[])
  n86 = Select(t=u8[] [] ("s? t:f"), s=w17, f=w15) -> (s? t:f=w4:u8[])
  "[Raw RxData]" <- w4
  n87 = feedback-in #1(w4) -> ()
  n88 = Index Array(array=w4) -> (element #3=w5:u8, element #4=w6:u8, element #5=w7:u8, element #6=w8:u8)  [unwired: 6 in, 2 out]
  n89 = Join Numbers(hi=w5, lo=w6) -> ((hi.lo)=w3:u16)
  n90 = Join Numbers(hi=w7, lo=w8) -> ((hi.lo)=w2:u16)
  n91 = Join Numbers(hi=w3, lo=w2) -> ((hi.lo)=→"DUT Serial Number":u32)
